vi "Actor.vi"(6 "Open Actor Core front panel? (F)":bool, 7 "error feedback":refnum<queue>, 9 "Actor":refnum<class "Actor.lvclass">, 10 "queue of queues":refnum<queue>, 11 "Message Enqueuer":refnum<class "Message Enqueuer.lvclass">) -> ()   [LabVIEW 2013, in "Actor Framework.lvlib" / "Actor.lvclass"]
doc: "(<B>Filename</B>: Actor Framework.lvlib:Actor.lvclass:Actor.vi)\n\nActor.vi is the top-level VI that is launched to be the functional aspect of the actor object. It is a wrapper around Actor Core.vi, which is where the actor defines most of its specific behavior. Actor.vi takes care of creating the caller-to-actor queue and brokering the exchange of enqueuers with the caller. It also handles all the cleanup when Actor Core.vi completes. It is not dynamic dispatch -- users of the actor framework generally don't need to understand what's being done in this function."
uses:
  <vilib>/ActorFramework/Actor/Actor.lvclass
  <vilib>/ActorFramework/Message Enqueuer/Message Enqueuer.lvclass
  <vilib>/ActorFramework/Message Enqueuer/Message Enqueuer.lvclass/Message Enqueuer.ctl
  <vilib>/ActorFramework/Actor/Actor.lvclass/Actor.ctl
  <vilib>/ActorFramework/Message/Message.lvclass
  <vilib>/ActorFramework/LastAck/Last Ack.lvclass/Last Ack.ctl
  <vilib>/ActorFramework/Message Enqueuer/Enqueue Critical.vi
  <vilib>/ActorFramework/Message Priority Queue/Priority Enqueue.vi
  <vilib>/ActorFramework/LastAck/Last Ack.lvclass
  <vilib>/ActorFramework/Message Priority Queue/Message Priority Queue.lvclass
panel:
  out "error out":errorcluster
  # "The error out is here only as an aid to debugging if necessary."
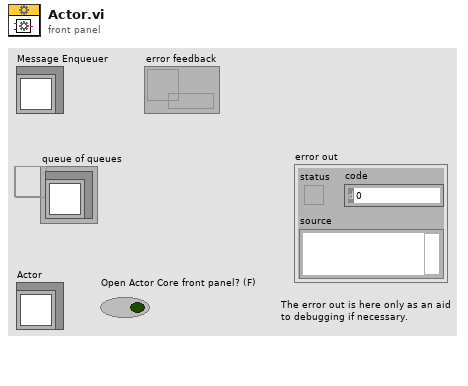
[diagram p1: front panel]
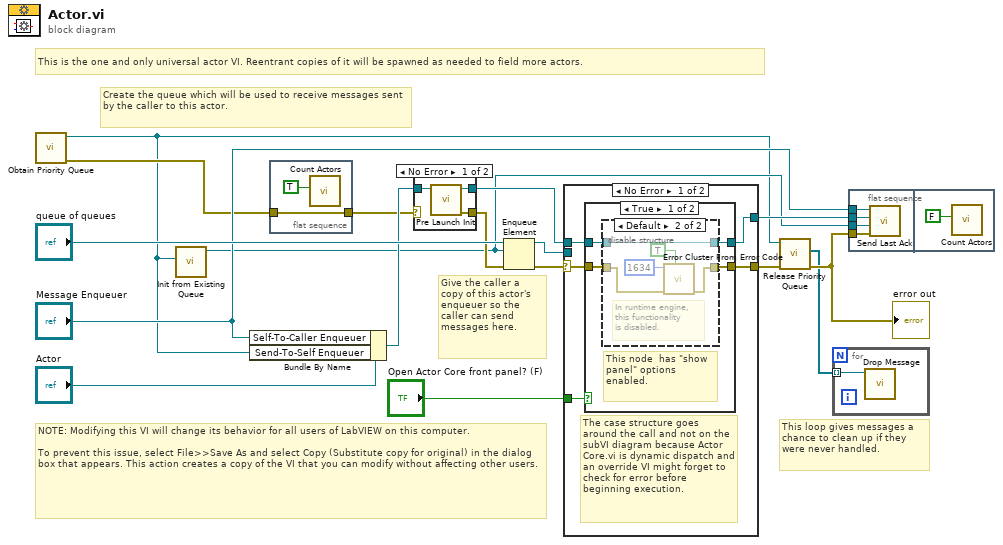
[diagram p0: block diagram]
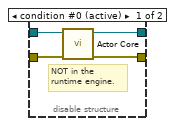
[diagram p3: hidden frame]
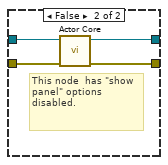
[diagram p4: hidden frame]
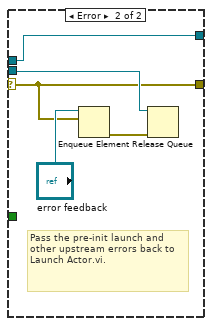
[diagram p5: hidden frame]
diagram:
  # "NOTE: Modifying this VI will change its behavior for all users of LabVIEW on this computer.\n\nTo prevent this issue, select File>>Save As and select Copy (Substitute copy for original) in the dialog box that appears. This action creates a copy of the VI that you can modify without affecting other users."
  # "This loop gives messages a chance to clean up if they were never handled."
  # "Give the caller a copy of this actor's enqueuer so the caller can send messages here."
  # "Create the queue which will be used to receive messages sent by the caller to this actor."
  # "This is the one and only universal actor VI. Reentrant copies of it will be spawned as needed to field more actors."
  n1 = call <vilib>:"Obtain Priority Queue.vi"() -> ("error out"=w3:errorcluster, "Priority Queue"=w1:refnum<class "Message Priority Queue.lvclass">)  [unwired: 10 in]
  n2 = call <vilib>:"Init from Existing Queue.vi"("Priority Queue"=w1) -> ("Message Enqueuer"=w2:refnum<class "Message Enqueuer.lvclass">)  [unwired: 10 in]
  n3 = Bundle By Name(cluster="Actor", "Self-To-Caller Enqueuer"="Message Enqueuer", "Send-To-Self Enqueuer"=w1) -> (w9:refnum<class "Actor.lvclass">)
  n4 = flat-sequence {
    tunnel: [w18] -> w4
    tunnel: w3 -> [w18]
    frame #0 {
      n5 = call <vilib>:"Count Actors.vi"("Increment?"=TRUE) -> ()  [unwired: 11 in]
    }
  }
  n6 = case shown="No Error" w4 {
    selector: w4 -> [_ w24]
    tunnel: w9 -> [w22 w23]
    tunnel: [w21 w23] -> w8
    tunnel: [w20 w24] -> w5
    frame No Error {
      n7 = call-dynamic "Pre Launch Init.vi"("Actor in"=w22) -> ("error out"=w20:errorcluster, "Actor out"=w21:refnum<class "Actor.lvclass">)  [unwired: 9 in]
    }
    frame Error {
    }
  }
  n8 = Enqueue Element(queue="queue of queues", element=w2, error in (no error)=w5) -> (queue out=w7:refnum<queue>, error out=w13:errorcluster)  [unwired: 1 in, 1 out]
  n9 = case shown="No Error" w13 {
    selector: w13 -> [w26 w47]
    tunnel: w8 -> [w27 w51]
    tunnel: [w29 w47] -> w17
    tunnel: [w28 w51] -> w15
    tunnel: w7 -> [_ w50]
    tunnel: "Open Actor Core front panel? (F)" -> [w25 _]
    frame No Error {
      # "The case structure goes around the call and not on the subVI diagram because Actor Core.vi is dynamic dispatch and an override VI might forget to check for error before beginning execution."
      n10 = case shown="True" w25 {
        tunnel: [w33 w46] -> w29
        tunnel: [w32 w45] -> w28
        tunnel: w27 -> [w31 w44]
        tunnel: w26 -> [w30 w43]
        frame True {
          # "This node  has \"show panel\" options enabled."
          n11 = disable-structure shown="Default" {
            disable-tunnel: [w37 w41] -> w33
            disable-tunnel: [w36 w42] -> w32
            disable-tunnel: w31 -> [w35 w42]
            disable-tunnel: w30 -> [w34 w40]
            frame condition #0 (active) {
              # "NOT in the \nruntime engine."
              n12 = call-dynamic "Actor Core.vi"("error in"=w34, "Actor in"=w35) -> ("error out"=w37:errorcluster, "Actor out"=w36:refnum<class "Actor.lvclass">)  [unwired: 8 in]
            }
            frame condition #1 {
              # "In runtime engine,\nthis functionality\nis disabled."
              n13 = call <vilib>:"Error Cluster From Error Code.vi"("show call chain? (False)"=TRUE, "error in (no error)"=w40, "error code (0)"=1634) -> ("error out"=w41:errorcluster)  [unwired: 6 in]
            }
          }
        }
        frame False {
          # "This node  has \"show panel\" options disabled."
          n14 = call-dynamic "Actor Core.vi"("error in"=w43, "Actor in"=w44) -> ("error out"=w46:errorcluster, "Actor out"=w45:refnum<class "Actor.lvclass">)  [unwired: 8 in]
        }
      }
    }
    frame Error {
      # "Pass the pre-init launch and other upstream errors back to Launch Actor.vi."
      n15 = Enqueue Element(queue="error feedback", element=w47) -> (error out=w48:errorcluster)  [unwired: 2 in, 2 out]
      n16 = Release Queue(queue=w50, error in (no error)=w48) -> ()  [unwired: 1 in, 3 out]
    }
  }
  n17 = call <vilib>:"Release Priority Queue.vi"("error in (no error)"=w17, "Priority Queue"=w1) -> ("error out"=w16:errorcluster, "remaining elements"=w12:refnum<class "Message.lvclass">[])  [unwired: 8 in]
  "error out" <- w16
  n18 = for {
    tunnel: w12 -> [w52] mode=indexing
    n19 = call <vilib>:"Drop Message.vi"("Message in"=w52) -> ()  [unwired: 11 in]
  }
  n20 = flat-sequence {
    tunnel: w16 -> [w56]
    tunnel: w15 -> [w55]
    tunnel: "Message Enqueuer" -> [w54]
    tunnel: w2 -> [w53]
    frame #0 {
      n21 = call <vilib>:"Send Last Ack.vi"("error from actor"=w56, "Caller-to-Actor Enqueuer"=w53, "Actor"=w55, "Message Enqueuer"=w54) -> ()  [unwired: 8 in]
    }
    frame #1 {
      n22 = call <vilib>:"Count Actors.vi"("Increment?"=FALSE) -> ()  [unwired: 11 in]
    }
  }
